vi "Test Base Card Passthrough (Properties).vi"() -> ()   [LabVIEW 2020, in "slsc-switch-benchmarks.lvlib"]
uses:
  slsc-switch-benchmarks.lvlib
panel:
  out "error out":errorcluster
  in  "Iterations":u32=1000
  in  "Channels to Sweep":i32=64
  out "#Channels Testing":i32
  out "Avg Connection Time":dbl(graph)
  in  "device":refnum<k21>="SET-2010-Mod2"
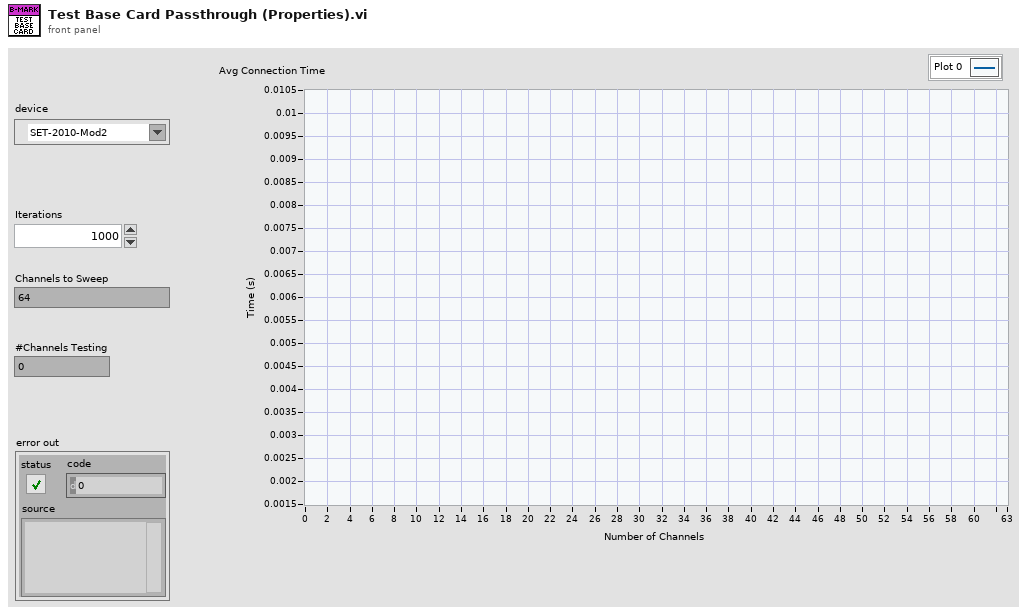
[diagram p1: front panel]
types:
  T1 = typedef "slsc-switch-benchmarks.lvlib/Timing Statistics.ctl" = cluster{"mean":dbl, "standard deviation":dbl, "maximum time":dbl, "minimum time":dbl}
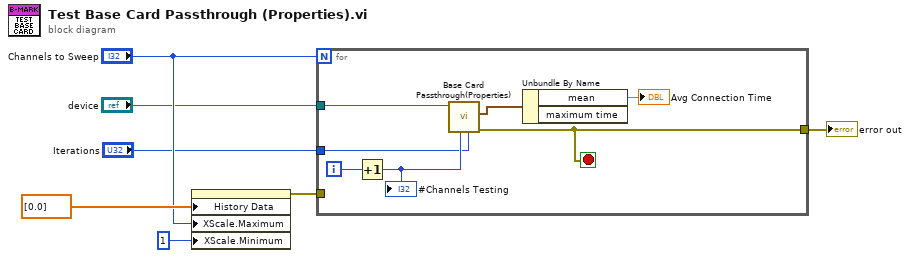
[diagram p0: block diagram]
diagram:
  n1 = property on="Avg Connection Time" class="WFChart (strict)"("History Data"=dbl[] [0.0], "XScale.Maximum"="Channels to Sweep", "XScale.Minimum"=1 ("Channels to Sweep")) -> (error out=w6:errorcluster)  [unwired: 2 in, 1 out]
  n2 = for {
    N: "Channels to Sweep" -> [_]
    tunnel: "device" -> [w13]
    tunnel: w6 -> [_]
    tunnel: "Iterations" -> [w11]
    tunnel: [w9] -> w1
    i -> [w14]
    stop <- w9 stop-if-true
    n3 = Increment(x=w14) -> (x+1=w12:i32)
    "#Channels Testing" <- w12
    n4 = call "Base Card Passthrough(Properties).vi"("Iterations"=w11, "Channels (1-64)"=w12, "device"=w13) -> ("error out"=w9:errorcluster, "Connect Timing"=w10:T1)  [unwired: 6 in, 1 out]
    n5 = Unbundle By Name(w10) -> ("mean"=→"Avg Connection Time":dbl)  [unwired: 1 out]
  }
  "error out" <- w1
